vi "Mutate Child Chromosome.vi"(10 "Mutation Rate":dbl, 11 "Child Chromosome In":refnum<class "IGene.lvclass">[](array[class])) -> (3 "Child Chromosome out":refnum<class "IGene.lvclass">[](array[class]))   [LabVIEW 2016, in "IPopulation.lvclass"]
uses:
  IPopulation/IPopulation.lvclass
  IGene/IGene.lvclass
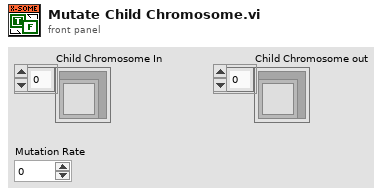
[diagram p1: front panel]
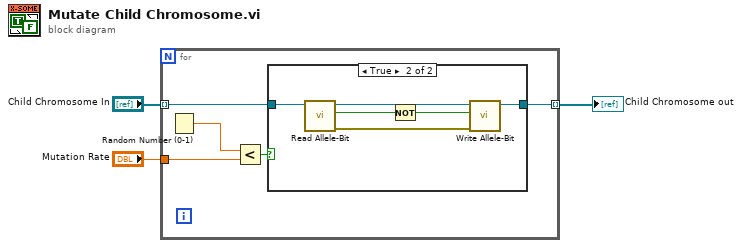
[diagram p0: block diagram]
diagram:
  n1 = for {
    tunnel: "Child Chromosome In" -> [w8] mode=indexing
    tunnel: [w5] -> w2 mode=indexing
    tunnel: "Mutation Rate" -> [w4]
    n2 = Random Number (0-1)() -> (number: 0 to 1=w7:dbl)
    n3 = Less?(x=w7, y=w4) -> (x < y?=w6:bool)
    n4 = case shown="True" w6 {
      tunnel: w8 -> [w9 w15]
      tunnel: [w9 w12] -> w5
      frame False {
      }
      frame True {
        n5 = call "Read Allele-Bit.vi"("IGene in"=w15) -> ("error out"=w10:errorcluster, "Allele-Bit"=w14:bool, "IGene out"=w13:refnum<class "IGene.lvclass">)  [unwired: 8 in]
        n6 = Not(x=w14) -> (.not. x?=w11:bool)
        n7 = call "Write Allele-Bit.vi"("error in (no error)"=w10, "Allele-Bit"=w11, "IGene in"=w13) -> ("IGene out"=w12:refnum<class "IGene.lvclass">)  [unwired: 7 in, 1 out]
      }
    }
  }
  "Child Chromosome out" <- w2
